vi "_Simulator SNA Tree.vi"   [LabVIEW 2011]
uses:
  SNA Command.ctl
panel:
  # "See Diagram"
types:
  T1 = typedef "SNA Command.ctl" = enum16{"LOAD", "INITIALIZE", "PRESET", "GET STIMULUS", "SET STIMULUS", "GET CALIBRATION", "CALIBRATE", "RESTORE", "MEASURE", "RELEASE", "UNLOAD", "CONFIRM", "SORT"}
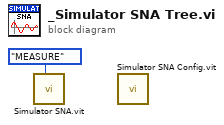
[diagram p0: block diagram]
diagram:
  n1 = call "Simulator SNA.vit"("SNA Command"=SNA_Command."MEASURE" ("VNA Command")) -> ()  [unwired: 5 in, 6 out]
  n2 = call "Simulator SNA Config.vit"() -> ()  [unwired: 2 in, 10 out]
